vi "FTW-XML-ValidateTagName.vi"(0 "Tag":string, 11 "error in":errorcluster) -> (4 "Valid Tag Name?":bool, 15 "error out":errorcluster)   [LabVIEW 2012]
uses:
  Error/FTW-ERR-ThrowError.vi
panel:
  # "Inputs"
  # "Outputs"
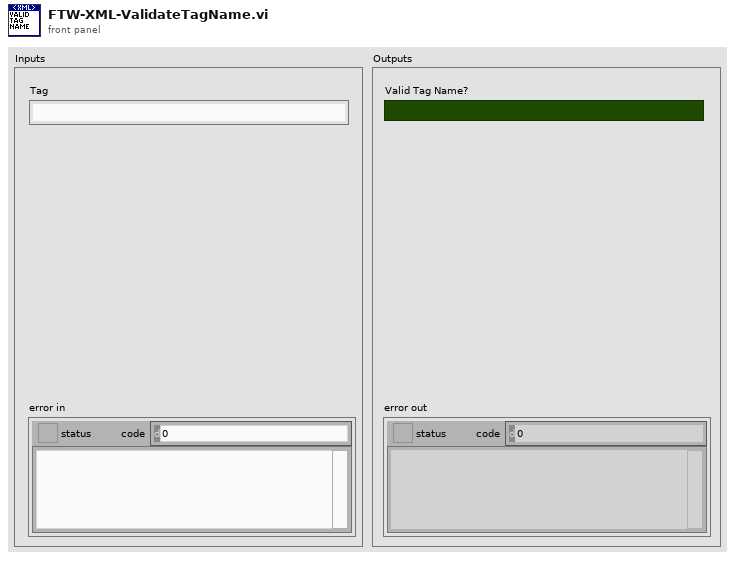
[diagram p1: front panel]
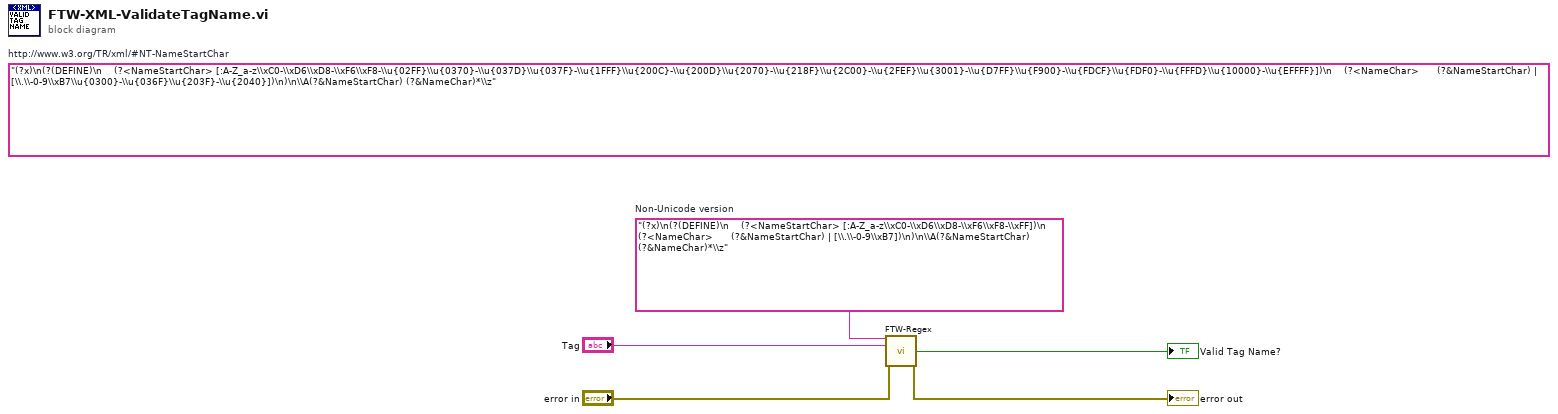
[diagram p0: block diagram]
diagram:
  (unwired) "(?x)\n(?(DEFINE)\n    (?<NameStartChar> [:A-Z_a-z\\xC0-\\xD6\\xD8-\\xF6\\xF8-\\u{02FF}\\u{0370}-\\u{037D}\\u{037F}-\\u{1FFF}\\u{200C}-\\u{200D}\\u{2070}-\\u{218F}\\u{2C00}-\\u{2FEF}\\u{3001}-\\u{D7FF}\\u{F900}-\\u{FDCF}\\u{FDF0}-\\u{FFFD}\\u{10000}-\\u{EFFFF}])\n    (?<NameChar>      (?&NameStartChar) | [\\.\\-0-9\\xB7\\u{0300}-\\u{036F}\\u{203F}-\\u{2040}])\n)\n\\A(?&NameStartChar) (?&NameChar)*\\z"  # http://www.w3.org/TR/xml/#NT-NameStartChar
  w1 = "(?x)\n(?(DEFINE)\n    (?<NameStartChar> [:A-Z_a-z\\xC0-\\xD6\\xD8-\\xF6\\xF8-\\xFF])\n    (?<NameChar>      (?&NameStartChar) | [\\.\\-0-9\\xB7])\n)\n\\A(?&NameStartChar) (?&NameChar)*\\z"  # Non-Unicode version
  n1 = call "FTW-Regex.vi"("Regular Expression"=w1, "Input String"="Tag", "error in"="error in") -> ("Match Found?"=→"Valid Tag Name?":bool, "error out"=→"error out":errorcluster)  [unwired: 8 in, 3 out]
